vi "RecordImages.vi"(0 "记录进度引用句柄":refnum<vi>, 1 "记录按钮引用句柄":refnum<vi>, 2 "输入图像":T1, 4 "记录路径引用句柄":refnum<vi>, 6 "记录帧数引用句柄":refnum<vi>, 8 "PacketSize":u32=1500, 9 "帧间隔/us":i64=200000 min=100000 max=500000 step=1, 10 "曝光时间(us)":i64, 11 "增益":i64=227) -> ()   [LabVIEW 2012]
uses:
  <vilib>/vision/Image Controls.llb/IMAQ Image.ctl
  <vilib>/Utility/xml.llb/Write to XML File.vi
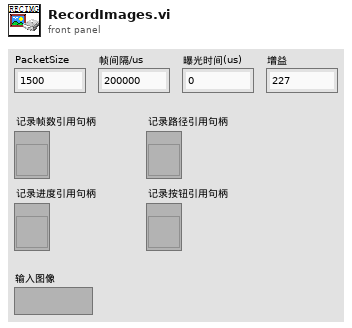
[diagram p1: front panel]
types:
  T1 = typedef "IMAQ Image.ctl" = refnum<image>
  T2 = enum8{"Enabled", "Disabled", "Disabled and Grayed Out"}
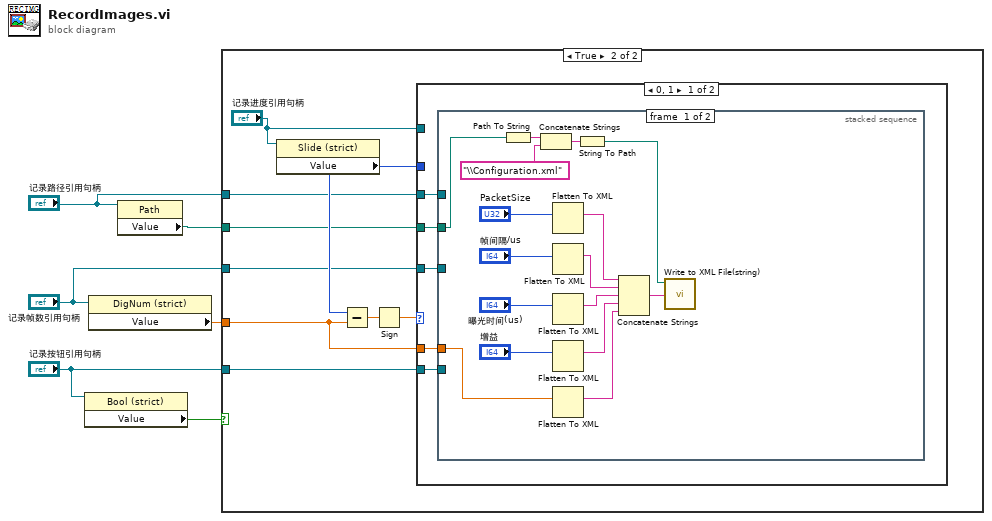
[diagram p0: block diagram]
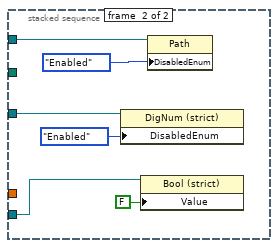
[diagram p3: hidden frame]
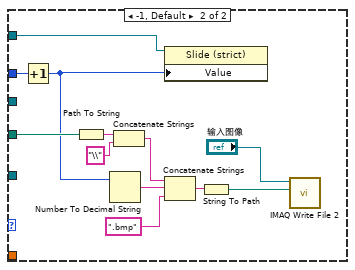
[diagram p4: hidden frame]
diagram:
  n1 = property class="Bool (strict)"(reference="记录按钮引用句柄") -> ("Value"=w6:bool)  [unwired: 1 in, 2 out]
  n2 = property class="DigNum (strict)"(reference="记录帧数引用句柄") -> ("Value"=w4:dbl)  [unwired: 1 in, 2 out]
  n3 = property class="Path"(reference="记录路径引用句柄") -> ("Value"=w3:path)  [unwired: 1 in, 2 out]
  n4 = case shown="True" w6 {
    tunnel: "记录按钮引用句柄" -> [_ w11]
    tunnel: w4 -> [_ w7]
    tunnel: w3 -> [_ w10]
    tunnel: "记录帧数引用句柄" -> [_ w9]
    tunnel: "记录路径引用句柄" -> [_ w8]
    frame False {
    }
    frame True {
      n5 = property class="Slide (strict)"(reference="记录进度引用句柄") -> ("Value"=w13:u8)  [unwired: 1 in, 2 out]
      n6 = Subtract(x=w13, y=w7) -> (x-y=w15:dbl)
      n7 = Sign(1:w15) -> (0:w14:dbl)
      n8 = case shown="0, 1" w14 {
        tunnel: w13 -> [_ w46]
        tunnel: "记录进度引用句柄" -> [_ w45]
        tunnel: w10 -> [w20 w44]
        tunnel: w11 -> [w19 _]
        tunnel: w9 -> [w18 _]
        tunnel: w8 -> [w17 _]
        tunnel: w7 -> [w16 _]
        frame 0, 1 {
          n9 = stacked-sequence {
            tunnel: w20 -> [w35 _]
            tunnel: w19 -> [_ w42]
            tunnel: w18 -> [_ w40]
            tunnel: w17 -> [_ w37]
            tunnel: w16 -> [w22 _]
            frame #0 {
              n10 = Path To String(path=w35) -> (string=w36:string)
              n11 = Concatenate Strings(w36, "\\Configuration.xml" ("字符串")) -> (w33:string)
              n12 = Flatten To XML(anything="PacketSize") -> (xml string=w27:string)
              n13 = Flatten To XML(anything="帧间隔/us") -> (xml string=w23:string)
              n14 = Flatten To XML(anything="曝光时间(us)") -> (xml string=w24:string)
              n15 = Flatten To XML(anything="增益") -> (xml string=w26:string)
              n16 = Flatten To XML(anything=w22) -> (xml string=w21:string)
              n17 = String To Path(string=w33) -> (path=w29:path)
              n18 = Concatenate Strings(w27, w23, w24, w26, w21) -> (w28:string)
              n19 = call-poly <vilib>:"Write to XML File(string).vi"("XML Input"=w28, "XML File Path"=w29) -> ()  [unwired: 3 in, 7 out]
            }
            frame #1 {
              n20 = property class="DigNum (strict)"(reference=w40, "DisabledEnum"=T2."Enabled" ("禁用")) -> ()  [unwired: 1 in, 2 out]
              n21 = property class="Bool (strict)"(reference=w42, "Value"=FALSE ("值")) -> ()  [unwired: 1 in, 2 out]
              n22 = property class="Path"(reference=w37, "DisabledEnum"=T2."Enabled" ("禁用")) -> ()  [unwired: 1 in, 2 out]
            }
          }
        }
        frame -1, Default {
          n23 = Increment(x=w46) -> (x+1=w43:u8)
          n24 = Path To String(path=w44) -> (string=w53:string)
          n25 = Number To Decimal String(number=w43) -> (decimal integer string=w50:string)  [unwired: 1 in]
          n26 = Concatenate Strings(w53, "\\" ("字符串")) -> (w49:string)
          n27 = property class="Slide (strict)"(reference=w45, "Value"=w43) -> ()  [unwired: 1 in, 2 out]
          n28 = Concatenate Strings(w49, w50, ".bmp" ("字符串")) -> (w51:string)
          n29 = String To Path(string=w51) -> (path=w48:path)
          n30 = call-poly "IMAQ Write File 2"("File Path"=w48, "Image"="输入图像") -> ()  [unwired: 8 in, 2 out]
        }
      }
    }
  }
